vi "Pcre2SubstringLengthByNumber8.vi"(8 "error in":errorcluster, 10 "Number":i32, 11 "pMatchData":u64 format="%.0x") -> (0 "error out":errorcluster, 1 "Length":u64, 2 "Number":i32, 3 "pMatchData":u64 format="%.0x")   [LabVIEW 2021, in "libpcre2-8.lvlib"]
uses:
  libpcre2-8.lvlib
  libpcre2-8-x32.dll
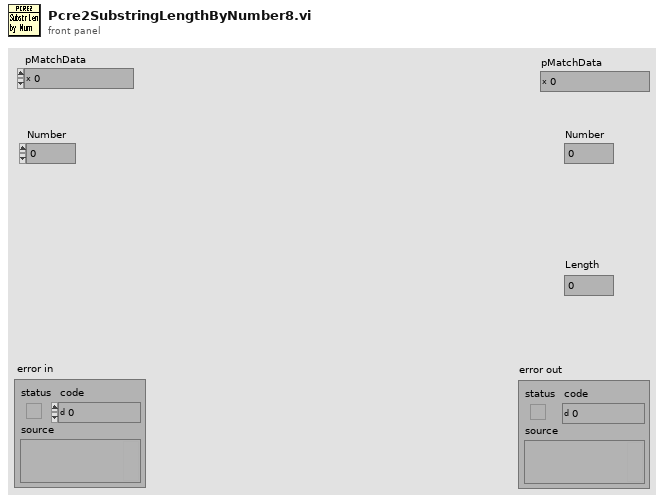
[diagram p1: front panel]
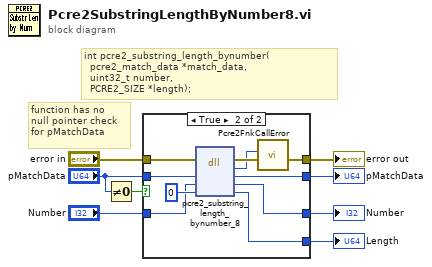
[diagram p0: block diagram]
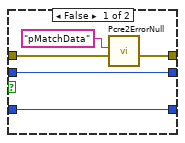
[diagram p2: hidden frame]
diagram:
  # "function has no \nnull pointer check \nfor pMatchData"
  # "int pcre2_substring_length_bynumber(\n  pcre2_match_data *match_data, \n  uint32_t number, \n  PCRE2_SIZE *length);"
  n1 = Not Equal To 0?(x="pMatchData") -> (x != 0?=w4:bool)
  n2 = case shown="True" w4 {
    tunnel: "error in" -> [w11 w22]
    tunnel: [w10 w15] -> w7
    tunnel: "pMatchData" -> [w13 w21]
    tunnel: [w13 w20] -> w6
    tunnel: [_ w18] -> w5
    tunnel: "Number" -> [w12 w19]
    tunnel: [w12 w17] -> w1
    frame False {
      n3 = call "Pcre2ErrorNull.vi"("error in"=w11, "What"="pMatchData" ("message")) -> ("error out"=w10:errorcluster)  [unwired: 9 in]
    }
    frame True {
      n4 = dll-call lib="libpcre2-8-x*.dll" fn="pcre2_substring_length_bynumber_8"(error in=w22, "match_data"=w21, "number"=w19, "length"=u64 0) -> (error out=w16:errorcluster, "return type"=w14:i32, "match_data"=w20:u64, "number"=w17:i32, "length"=w18:u64)  [unwired: 2 in, 1 out]
      n5 = call "Pcre2FnkCallError.vi"("error in"=w16, "ErrorCode"=w14) -> ("error out"=w15:errorcluster)  [unwired: 9 in]
    }
  }
  "pMatchData" <- w6
  "error out" <- w7
  "Length" <- w5
  "Number" <- w1
